vi "play_auto_id.vi"(3 "output-file":path=path "C:/Users/arnold/Documents/afm-cs/labview/first_res_fit_current.json", 4 "time-series-in":refnum<vi>, 6 "Bode amplitude_in":refnum<vi>, 8 "error in":errorcluster, 10 "Amplitude":dbl=0.1 format="%#_13g", 11 "Swept-Sines-Control-Settings":cluster{"u-max":sgl, "offset":sgl, "Ki":sgl}={"u-max"=1.0, "offset"=0.1, "Ki"=0.0}) -> (0 "error out":errorcluster, 1 "Is-Totally-Stable":bool, 2 "auto_id_result":T1)   [LabVIEW 2017]
uses:
  controls/SS_SweptSines.ctl
  controls/SS_sin_params.ctl
  controls/SS_input_data_json.ctl
  controls/fit_sos_results.ctl
  controls/auto_id_result.ctl
  controls/SOS_frf_data.ctl
  controls/logging_selection.ctl
  controls/SS_figures_withtime.ctl
  controls/bode_figure.ctl
  labview/sysID/controls/time_series_figures.ctl
  <vilib>/Utility/error.llb/DialogType.ctl
  <vilib>/FPGAPlugInAG/cRIO-9082/niLvFpga_Open_cRIO-9082.vi
  <vilib>/rvi/interface/common/dynamic/niFpgaDynamicAddResources.vi
  <vilib>/FPGAPlugInAG/Dynamic/niLvFpga_Reset_Dynamic.vi
  <vilib>/rvi/interface/common/niFpgaWaitOnOcc.vi
  <vilib>/Utility/error.llb/Error Cluster From Error Code.vi
  <vilib>/rvi/errors/niLvFpgaAdjustHostInterfaceError.vi
  <vilib>/FPGAPlugInAG/Dynamic/niLvFpga_Run_Dynamic.vi
  <vilib>/FPGAPlugInAG/Dynamic/niLvFpga_Close_Dynamic.vi
  <vilib>/rvi/interface/nirviOpenFPGA/nirviOpenFPGA.xnode
  FPGA Bitfiles/afmimagingcontro_FPGATargetSPARTA_SSfpgasweptsines_lpZqvyn1KNg.lvbitx
  <vilib>/rvi/interface/nirviMethod/nirviMethod.xnode
  <vilib>/rvi/interface/nirviReadWriteControl/nirviReadWriteControl.xnode
  <vilib>/rvi/interface/nirviCloseFPGA/nirviCloseFPGA.xnode
  labview/utils_lib/utils.lvlib
  NiFpgaLv.dll
  <vilib>/rvi/interface/Simulation/niFpgaSimulationCallBeginRW.vi
  <vilib>/addons/_JKI.lib/Serialization/JSON/JKI JSON Serialization.lvlib
  <vilib>/FPGAPlugInAG/Dynamic/niLvFpga_ConfigureFifo_Dynamic.vi
  <vilib>/rvi/errors/niLvFpgaMergeErrorWithErrorCode.vi
panel:
  in  "Tab Control":enum32{"Page 1", "debug", "hide"}(tab)
  in  "control-xy-to-zero":bool=TRUE
  in  "ABORT":bool
  out "fit_sos_result":T3
  in  "theta0":dbl[](array[numeric])=[0.6786, -1.9959, 0.99891, -1.996142, 0.9989]
  out "theta-fit":dbl[](array[numeric])
  out "Bode amplitude":cluster{"W":dbl[], "Magnitude":dbl[]}[](graph) caption="Magnitude Graph"
  in  "Input File (json)":path=path "Z:/afm-cs/sysID/z-axis_sines_info_quick_firstRes.json"
  in  "Figures":enum32{"all-channels", "channel-1", "channel2"}(tab)
  out "Channel 1":cluster{"W":dbl[], "Magnitude":dbl[]}[](graph) caption="Magnitude Graph"
  in  "subtract-mean":bool=TRUE
  out "Channel1 2":cluster{"W":dbl[], "Phase":dbl[]}[](graph) caption="Phase Graph"
  out "Channel 3":cluster{"W":dbl[], "Magnitude":dbl[]}[](graph) caption="Magnitude Graph"
  out "boolean  indicators":T4
  out "Freqs Done":i32(slide) scale=0.0..50.0
  out "number_of_freqs":i32
  out "freq_adjusted":dbl
  out "NaN/Path/Refnum?":bool
  in  "SweptSines (in)":T5={"Log-Channel_select"=[FALSE, FALSE, FALSE, FALSE, FALSE, FALSE], "JSON Header"="", "SS-Params-Array"=[], "input_frequency_definitions"={"Amp"=0.0, "Ts"=0.0, "num_periodsMT"=[], "freqs_Hz"=[], "numAve_s"=[], "Nsamp_total"=[], "Nsettle_s"=[], "Ncollect_s"=[]}, "DAC-ADC primary 2"=0, "Channel-Names"=[], "num_chan"=0, "num-freqs"=0, "Input File (json)"=path "Z:/afm-cs/sysID/x-axis_sines_info_intsamps_quick.json"} {"DAC-ADC primary 2" items=["DAC0/ADC0", "DAC1/ADC1", "DAC2/ADC2", "DAC3/ADC3", ""]}
  out "TsTicks":u32
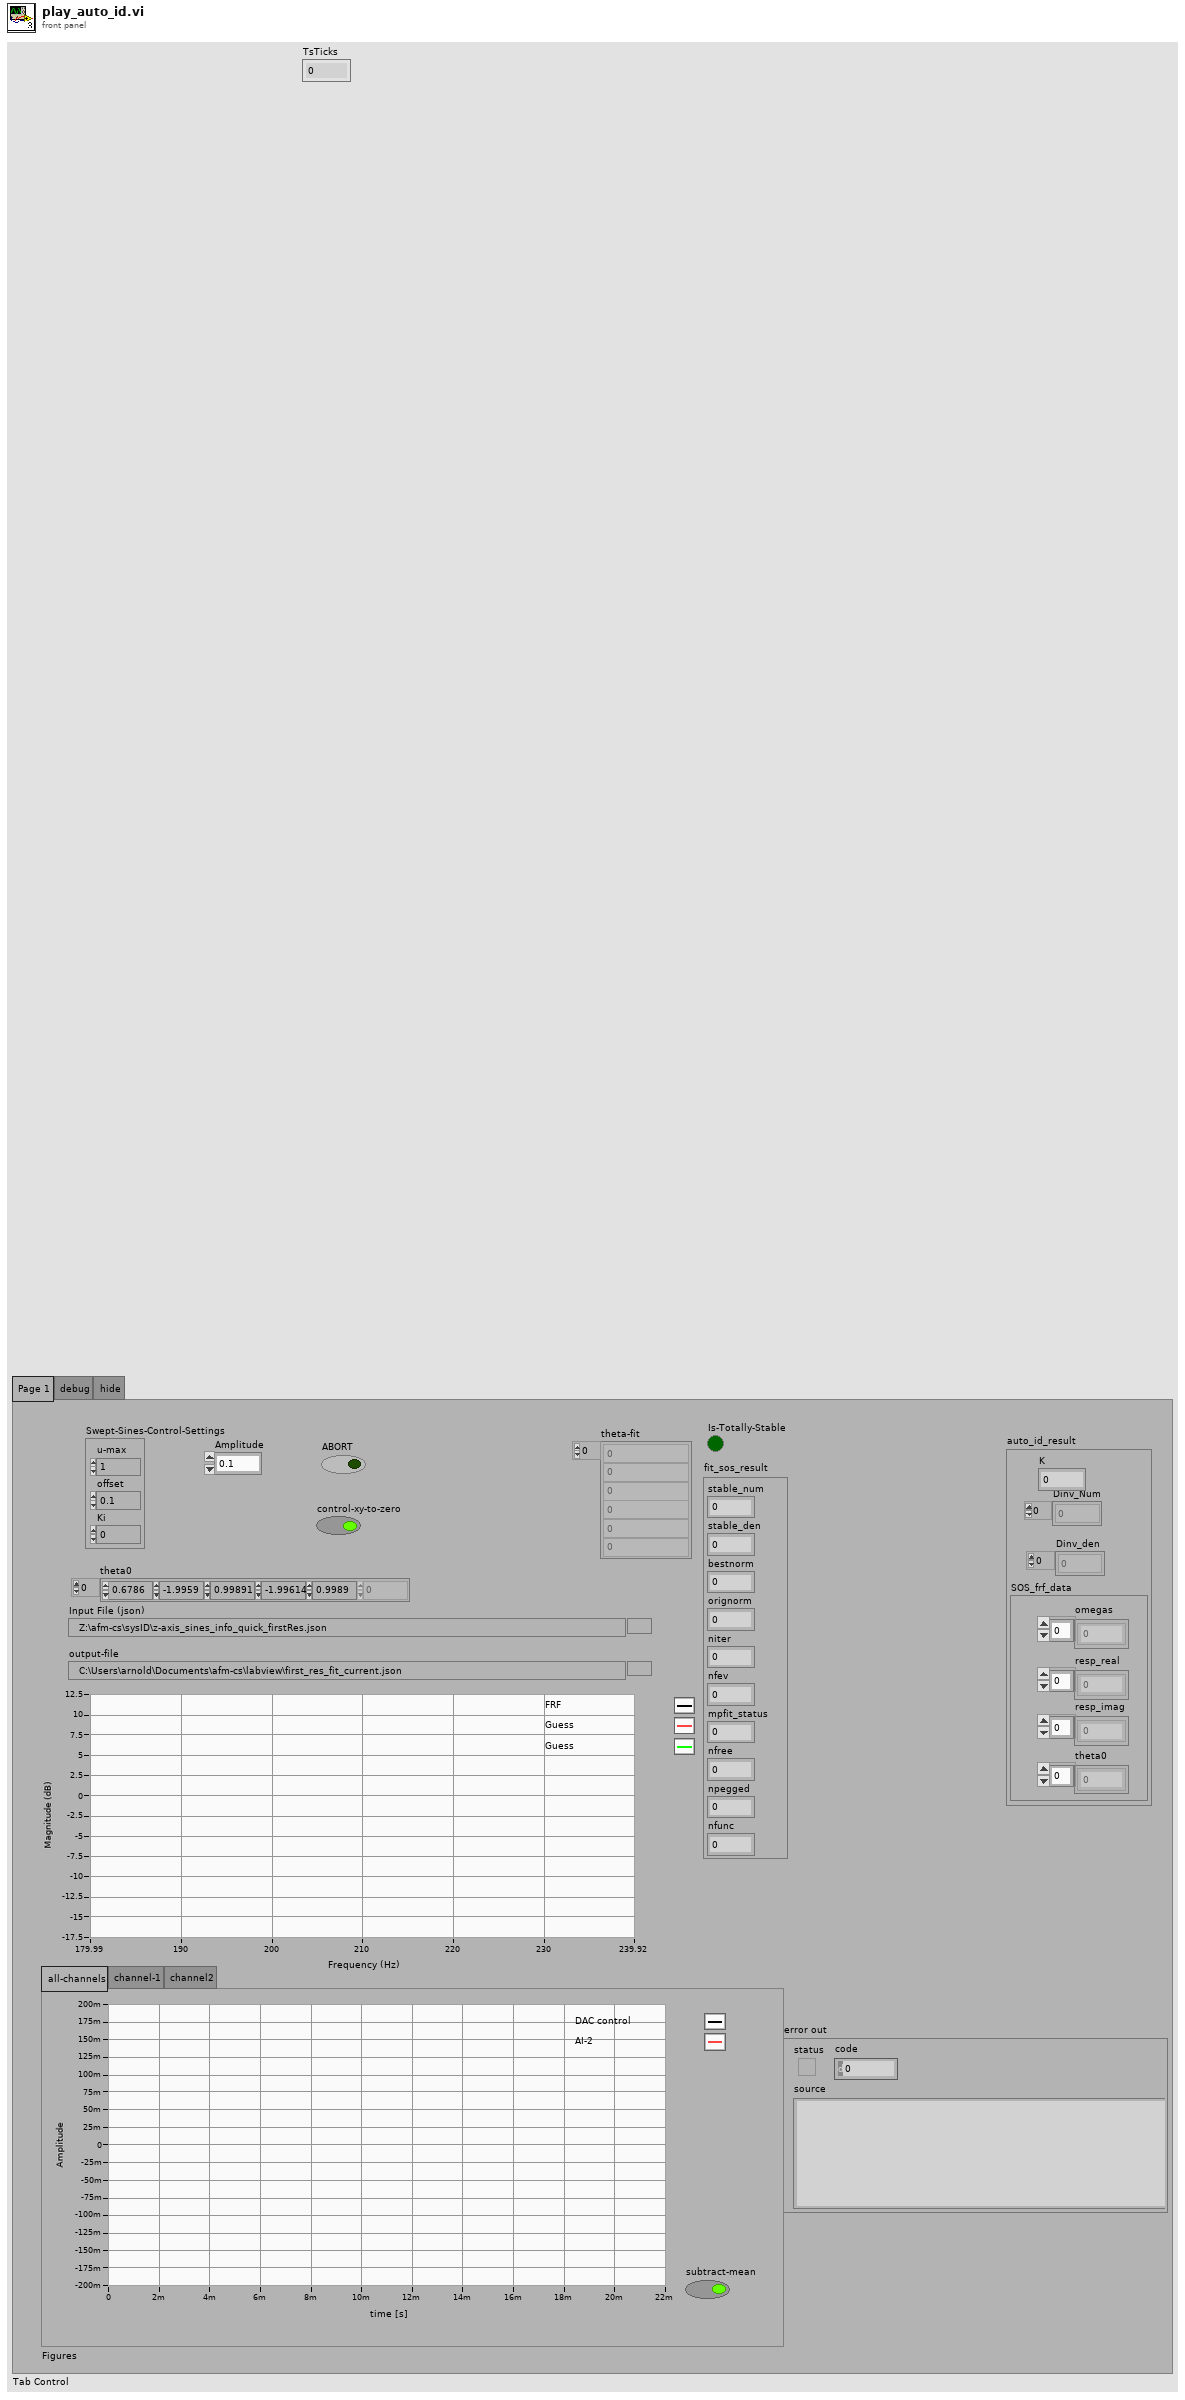
[diagram p1: front panel]
types:
  T1 = typedef "auto_id_result.ctl" = cluster{"Dinv_Num":dbl[], "SOS_frf_data":T2, "Dinv_den":dbl[], "K":dbl}
  T2 = typedef "SOS_frf_data.ctl" = cluster{"omegas":dbl[], "resp_real":dbl[], "resp_imag":dbl[], "theta0":dbl[]}
  T3 = typedef "fit_sos_results.ctl" = cluster{"stable_num":i32, "stable_den":i32, "bestnorm":dbl, "orignorm":dbl, "niter":i32, "nfev":i32, "mpfit_status":i32, "nfree":i32, "npegged":i32, "nfunc":i32}
  T4 = cluster{"unstable-z-traj":bool, "input fifo time-out":bool, "logging fifo timeout":bool, "scanning finished":bool, "unstable-x-traj":bool, "unstable-y-traj":bool, "ABORT":bool, "All Measurements Done":bool, "fpga_finished":bool, "current_scan_finished":bool}
  T5 = typedef "SS_SweptSines.ctl" = cluster{"Log-Channel_select":bool[], "JSON Header":string, "SS-Params-Array":T6[], "input_frequency_definitions":T7, "DAC-ADC primary 2":i16, "Channel-Names":string[], "num_chan":i32, "num-freqs":i32, "Input File (json)":path}
  T6 = typedef "SS_sin_params.ctl" = cluster{"freq":dbl, "num_samples":i32, "Amp":dbl, "Ts":dbl, "N_settle":u32, "Ncollect":i32, "num_periodsMT":i32, "num_averages":i32}
  T7 = typedef "SS_input_data_json.ctl" = cluster{"Amp":dbl, "Ts":dbl, "num_periodsMT":u32[], "freqs_Hz":dbl[], "numAve_s":i32[], "Nsamp_total":u32[], "Nsettle_s":u32[], "Ncollect_s":u32[]}
  T8 = typedef "SS_figures_withtime.ctl" = cluster{"bode figures":T9, "time-series figures":T10, "Freqs Done":refnum<vi>}
  T9 = typedef "bode_figure.ctl" = cluster{"Bode phase":refnum<vi>, "Bode amplitude":refnum<vi>}
  T10 = typedef "time_series_figures.ctl" = refnum<vi>[]
  T11 = typedef "logging_selection.ctl" = cluster{"Collect reference":bool, "Collect DAC control":bool, "Collect AI-0":bool, "Collect AI-1":bool, "Collect AI-2":bool, "Collect AI-3":bool}
  T12 = typedef "FrdData.ctl" = cluster{"Frequency Unit":enum16{"Hz", "rad/s"}, "W":dbl[], "MagDB":dbl[], "PhaseDeg":dbl[], "Resp":cdb[], "Data-name":string}
  T13 = typedef "DialogType.ctl" = u16
  T14 = typedef "SS_experimental-data.ctl" = cluster{"sin-data-out":dbl[][], "Fourier Data":T15, "freq_adjusted?":dbl, "below-nyquist":bool}
  T15 = typedef "SS_FourierData.ctl" = cluster{"E_s":dbl[], "Fourier Coefs":cdb[], "freq-adjusted":dbl}
  T16 = enum16{"open", "replace", "create", "open or create", "replace or create", "replace or create with confirmation"}
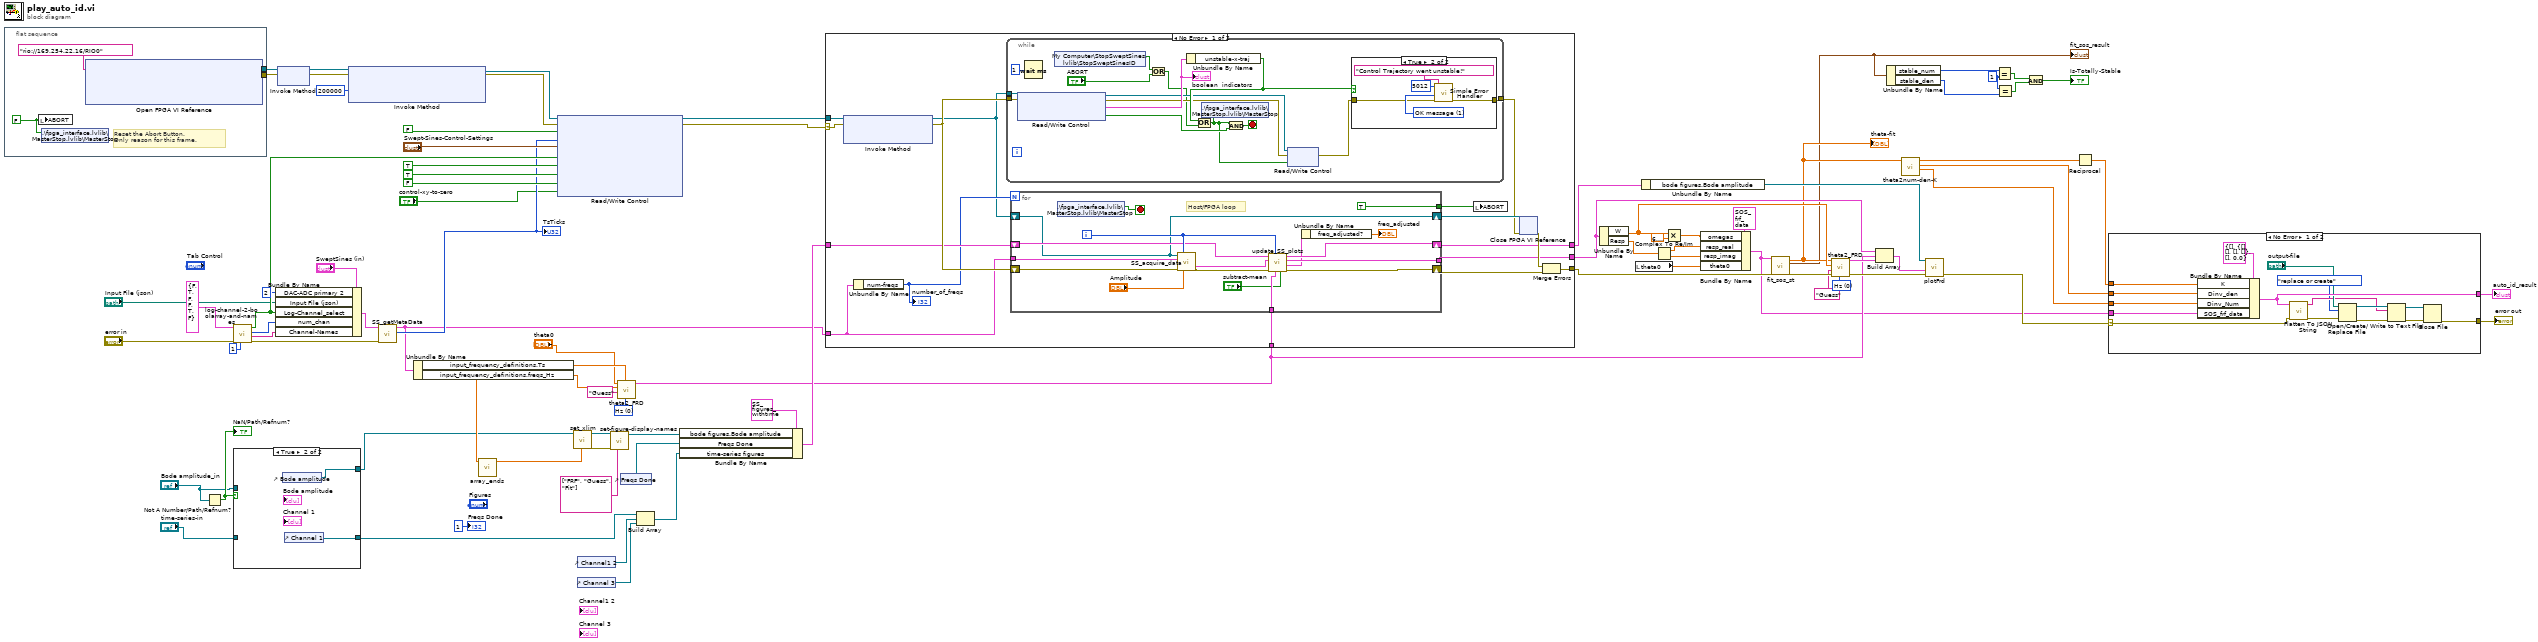
[diagram p0: block diagram]
diagram:
  w23 = 1
  w48 = u16 0 items=["Hz", "rad/s"] ("freq unit")
  w56 = u16 0 items=["Hz", "rad/s"] ("freq unit")
  n1 = flat-sequence {
    tunnel: [w88] -> w84
    tunnel: [w87] -> w83
    frame #0 {
      w86 = FALSE
      # "Reset the Abort Button.\nOnly reason for this frame."
      n2 = local write "ABORT"(w86) -> ()
      n3 = shared-variable ".\\fpga_interface.lvlib\\MasterStop.lvlib\\MasterStop"(w86) -> ()  [unwired: 1 in, 1 out]
      n4 = xnode "Open FPGA VI Reference"("resource name"=tag "rio://169.254.22.16/RIO0") -> ("FPGA VI Reference Out"=w88:refnum<k20>, "error out"=w87:errorcluster)  [unwired: 1 in]
    }
  }
  n5 = Not A Number/Path/Refnum?(number/path/refnum="Bode amplitude_in") -> (NaN/Path/Refnum?=w5:bool)
  "NaN/Path/Refnum?" <- w5
  n6 = call "log-channel-2-boolarray-and-names.vi"("min_number_chan"=i16 1, "error in"="error in", "Logging selection"=T11 {"Collect reference"=FALSE, "Collect DAC control"=TRUE, "Collect AI-0"=FALSE, "Collect AI-1"=FALSE, "Collect AI-2"=TRUE, "Collect AI-3"=FALSE}) -> ("error out"=w72:errorcluster, "Channel-Names"=w70:string[], "num_chan"=w67:i32, "Log-Channel_select"=w65:bool[])  [unwired: 5 in]
  n7 = case shown="True" w5 {
    tunnel: [w91 w93] -> w3
    tunnel: "Bode amplitude_in" -> [w91 _]
    tunnel: [w90 w92] -> w2
    tunnel: "time-series-in" -> [w90 _]
    frame False {
    }
    frame True {
      n8 = control-ref of="Bode amplitude"() -> (w93:refnum<vi>)
      n9 = control-ref of="Channel 1"() -> (w92:refnum<vi>)
    }
  }
  n10 = Bundle By Name(cluster="SweptSines (in)", "DAC-ADC primary 2"=i16 2, "Input File (json)"="Input File (json)", "Log-Channel_select"=w65, "num_chan"=w67, "Channel-Names"=w70) -> (w69:T5)
  n11 = xnode "Invoke Method"("FPGA VI Reference In"=w84, "error in"=w83) -> ("FPGA VI Reference Out"=w77:refnum<k20>, "error out"=w76:errorcluster)
  n12 = xnode "Invoke Method"("FPGA VI Reference In"=w77, "error in"=w76, "Requested Depth"=200000 ("requested depth")) -> ("FPGA VI Reference Out"=w82:refnum<k20>, "error out"=w78:errorcluster)  [unwired: 1 out]
  n13 = call "SS_getMetaData.vi"("error in"=w72, "SweptSines"=w69) -> ("TsTicks"=w62:u32, "SweptSines (out)"=w33:T5)  [unwired: 6 in, 1 out]
  "TsTicks" <- w62
  n14 = Unbundle By Name(w33) -> ("input_frequency_definitions.Ts"=w55:dbl, "input_frequency_definitions.freqs_Hz"=w54:dbl[])
  n15 = call "array_ends.vi"("freqs_Hz"=w54) -> ("Array"=w58:dbl[])  [unwired: 10 in]
  n16 = xnode "Read/Write Control"("FPGA VI Reference In"=w82, "error in"=w78, "ABORT"=FALSE, "TsTicks"=w62, "Swept-Sines-Control-Settings"="Swept-Sines-Control-Settings", "Log-Channel_select"=w65, "Subtract y0?"=TRUE ("Subtract-origin"), "reset"=TRUE, "Close Loop?"=FALSE, "control-xy-zero"="control-xy-to-zero") -> ("FPGA VI Reference Out"=w74:refnum<k20>, "error out"=w73:errorcluster)
  n17 = call "set_xlim.vi"("xlim"=w58, "figure (in)"=w3) -> ("error out"=w59:errorcluster, "figure (out)"=w60:refnum<vi>)  [unwired: 8 in]
  n18 = control-ref of="Channel1 2"() -> (w8:refnum<vi>)
  n19 = control-ref of="Channel 3"() -> (w7:refnum<vi>)
  n20 = call "set-figure-display-names.vi"("DisplayNames"=string[] ["FRF", "Guess", "Fit"] ("Data_names"), "error in"=w59, "figure (in)"=w60) -> ("figure (out)"=w53:refnum<vi>)  [unwired: 7 in, 1 out]
  n21 = call "theta2_FRD.vi"("freq unit"=w56, "Sampling Time (s)"=w55, "Data-name"="Guess", "freqs/omega"=w54, "theta"="theta0") -> ("FRD-model"=w34:T12)  [unwired: 5 in, 1 out]
  n22 = control-ref of="Freqs Done"() -> (w29:refnum<vi>)
  n23 = Build Array(w2, w8, w7) -> (w6:refnum<vi>[])
  n24 = Bundle By Name(cluster=T8 {"bode figures"={"Bode phase"=refnum, "Bode amplitude"=refnum}, "time-series figures"=[], "Freqs Done"=refnum} ("figures"), "bode figures.Bode amplitude"=w53, "Freqs Done"=w29, "time-series figures"=w6) -> (w52:T8)
  n25 = case shown="No Error" w73 {
    selector: w73 -> [w99 w149]
    tunnel: w74 -> [w109 _]
    tunnel: [w104 w149] -> w61
    tunnel: w33 -> [w101 _]
    tunnel: w52 -> [w102 w148]
    tunnel: [w97 w148] -> w40
    tunnel: w34 -> [w96 _]
    tunnel: [w95 _] -> w35
    frame No Error {
      n26 = xnode "Invoke Method"("FPGA VI Reference In"=w109, "error in"=w99) -> ("FPGA VI Reference Out"=w94:refnum<k20>, "error out"=w107:errorcluster)  [unwired: 1 in]
      n27 = Unbundle By Name(w101) -> ("num-freqs"=w100:i32)
      "number_of_freqs" <- w100
      n28 = while {
        tunnel: w94 -> [w123]
        tunnel: w107 -> [w122]
        tunnel: [w119] -> w103
        stop <- w115 stop-if-true
        n29 = xnode "Read/Write Control"("FPGA VI Reference In"=w123, "error in"=w122) -> ("FPGA VI Reference Out"=w118:refnum<k20>, "error out"=w117:errorcluster, "boolean  indicators"=w121:T4, "All Done"=w114:bool)
        "boolean  indicators" <- w121
        n30 = Wait (ms)(milliseconds to wait=u32 1) -> ()  [unwired: 1 out]
        n31 = shared-variable "My Computer\\StopSweptSines.lvlib\\StopSweptSinesID"() -> (w110:bool)  [unwired: 1 in, 1 out]
        n32 = Or(x=w110, y="ABORT") -> (x .or. y?=w111:bool)
        n33 = Unbundle By Name(w121) -> ("unstable-x-traj"=w120:bool)
        n34 = Or(x=w120, y=w111) -> (x .or. y?=w113:bool)
        n35 = shared-variable ".\\fpga_interface.lvlib\\MasterStop.lvlib\\MasterStop"(w113) -> ()  [unwired: 1 in, 1 out]
        n36 = And(x=w113, y=w114) -> (x .and. y?=w115:bool)
        n37 = xnode "Read/Write Control"("FPGA VI Reference In"=w118, "error in"=w117, "ABORT"=w113) -> ("error out"=w116:errorcluster)  [unwired: 1 out]
        n38 = case shown="True" w120 {
          tunnel: w116 -> [w125 w127]
          tunnel: [w125 w126] -> w119
          frame False {
          }
          frame True {
            w130 = T13 1 items=["no dialog", "OK message", "continue or stop message", "OK message + warnings", "continue/stop + warnings"] ("type of dialog (OK msg:1)")
            n39 = call <vilib>:"Simple Error Handler.vi"("error code (no error:0)"=5012, "error source (\" \")"="Control Trajectory went unstable!" ("error source (\" \")"), "type of dialog (OK msg:1)"=w130, "error in (no error)"=w127) -> ("error out"=w126:errorcluster)  [unwired: 1 in, 4 out]
          }
        }
      }
      n40 = for {
        N: w100 -> [_]
        shift-right: [w137] -> w97
        shift-left: w102 -> [w136]
        tunnel: [TRUE] -> w106
        shift-right: [w143] -> w98
        shift-left: w107 -> [w145]
        tunnel: w101 -> [w144]
        tunnel: [w138] -> w95
        tunnel: w96 -> [w134]
        shift-right: [w132] -> w108
        shift-left: w94 -> [w132]
        i -> [w141]
        stop <- w133 stop-if-true
        # "Host/FPGA loop"
        n41 = shared-variable ".\\fpga_interface.lvlib\\MasterStop.lvlib\\MasterStop"() -> (w133:bool)  [unwired: 1 in, 1 out]
        n42 = call "SS_acquire_data.vi"("Type"=w132, "idx"=w141, "SweptSines (in)"=w144, "error in"=w145, "Signal Amplitude (V)"="Amplitude") -> ("experiment-data"=w140:T14, "error IO"=w139:errorcluster)  [unwired: 7 in, 2 out]
        n43 = call "update_SS_plots.vi"("subtract-mean"="subtract-mean", "other-frd"=w134, "freqs-iter"=w141, "error in (no error)"=w139, "experiment-data"=w140, "figures-in"=w136) -> ("error out"=w143:errorcluster, "experiment-data (out)"=w135:T14, "FRD-out"=w138:T12, "figures-out"=w137:T8)  [unwired: 2 in]
        n44 = Unbundle By Name(w135) -> ("freq_adjusted?"=→"freq_adjusted":dbl)
      }
      n45 = local write "ABORT"(w106) -> ()
      n46 = xnode "Close FPGA VI Reference"("FPGA VI Reference In"=w108, "error in"=w103) -> ("error out"=w105:errorcluster)
      n47 = Merge Errors(w105, w98) -> (w104:errorcluster)
    }
    frame Error {
    }
  }
  n48 = Unbundle By Name(w35) -> ("W"=w28:dbl[], "Resp"=w42:cdb[])
  n49 = local read "theta0"() -> (w41:dbl[])
  n50 = Unbundle By Name(w40) -> ("bode figures.Bode amplitude"=w36:refnum<vi>)
  n51 = Complex To Re/Im(x + iy=w42) -> (x=w44:dbl[], y=w43:dbl[])
  n52 = Multiply(x=w28, y=6.283185307179586) -> (x*y=w46:dbl[])
  n53 = Bundle By Name(cluster=T2 {"omegas"=[1006.674891, 1016.262272, 1025.849652, 1035.437033, 1045.024413, 1054.611794, 1064.199174, 1073.786548, 1083.373929, 1092.961309, 1102.54869, 1112.13607, 1121.723451, 1131.310831, 1140.898212, 1150.485592, 1160.072973, 1169.660354, 1179.247728, 1188.835108, 1198.422489, 1208.009869, 1217.59725, 1227.18463, 1236.772011, 1246.359391, 1255.946772, 1265.534152, 1275.121533, 1284.708907, 1294.296288, 1303.883668, 1313.471049, 1323.058429, 1332.64581, 1342.23319, 1351.820571, 1361.407951, 1370.995332, 1380.582706, 1390.170086, 1399.757467, 1409.344847, 1418.932228, 1428.519609, 1438.106989, 1447.69437, 1457.28175, 1466.869131, 1476.456511, 1486.043885, 1495.631266, 1505.218646, 1514.806027, 1524.393407, 1533.980788, 1543.568168, 1553.155549, 1562.742929, 1572.33031, 1581.91769, 1591.505065, 1601.092445, 1610.679826, 1620.267206, 1629.854587, 1639.441967, 1649.029348, 1658.616728], "resp_real"=[0.6710936201, 0.6732167298, 0.6736550301, 0.6739624194, 0.6764113406, 0.6760996891, 0.6752809587, 0.67695858, 0.6764911126, 0.6818501379, 0.6804259731, 0.6777421689, 0.683602427, 0.6839502494, 0.6873055899, 0.6871681129, 0.6836241729, 0.6933718335, 0.6965190689, 0.7011525702, 0.7041006273, 0.7087951209, 0.7138881005, 0.7230810664, 0.7347158563, 0.743593779, 0.7581554602, 0.7740064901, 0.7983882262, 0.8168799192, 0.8500537495, 0.885993569, 0.8534751304, 0.6135298299, 0.1963078728, 0.06997493602, 0.2143720387, 0.3262401307, 0.3874363268, 0.4244315327, 0.4518076771, 0.4783094111, 0.4942330365, 0.5078067569, 0.5183774173, 0.5254372068, 0.5346584888, 0.5422376, 0.5476692529, 0.546204086, 0.5501300272, 0.5526801006, 0.557631838, 0.5639162136, 0.5601299408, 0.5627301292, 0.5646599194, 0.5678509651, 0.5674161925, 0.5676099823, 0.5703128211, 0.5717199117, 0.5717616028, 0.5714305364, 0.5706488864, 0.574491682, 0.5720673373, 0.5722619255, 0.5727540208], "resp_imag"=[0.1828230252, 0.185702312, 0.1893108783, 0.1927179342, 0.1939516982, 0.1991804891, 0.1996588255, 0.1997489381, 0.2009184192, 0.2058333084, 0.205968755, 0.2071290225, 0.2120033665, 0.2140896781, 0.2197333799, 0.2218060221, 0.2270970718, 0.2243543787, 0.2282290931, 0.2349554807, 0.2362899955, 0.2386023634, 0.2479762836, 0.2514213949, 0.2589829258, 0.2690734156, 0.2817668466, 0.3075000844, 0.3292949756, 0.3581777586, 0.418098085, 0.518537997, 0.7274335428, 0.9954410219, 0.8283414758, 0.4651799029, 0.2632646215, 0.2204933474, 0.2100370796, 0.215817828, 0.2094899805, 0.2041701149, 0.2090161752, 0.2122336611, 0.2144513636, 0.2154505064, 0.2184072105, 0.2207006189, 0.2264320741, 0.2319746485, 0.2352243002, 0.2359211056, 0.2344839067, 0.234200787, 0.2350554818, 0.2419460399, 0.2451480379, 0.2422561944, 0.2450402058, 0.2520603413, 0.2526693987, 0.2530329194, 0.2523935129, 0.2570623818, 0.2576871444, 0.2563998974, 0.259830217, 0.2610581842, 0.2647075477], "theta0"=[0.6786, -1.9959, 0.99891, -1.996142, 0.9989]} ("SOS-frf_data"), "omegas"=w46, "resp_real"=w44, "resp_imag"=w43, "theta0"=w41) -> (w16:T2)
  n54 = call "fit_sos_st.vi"("frf_data"=w16, "error in (no error)"=w61) -> ("theta"=w27:dbl[], "fit_sos_result"=w26:T3, "error out"=w50:errorcluster)  [unwired: 23 in]
  "fit_sos_result" <- w26
  "theta-fit" <- w27
  n55 = call "theta2_FRD.vi"("freq unit"=w48, "error in (no error)"=w50, "Data-name"="Guess", "freqs/omega"=w28, "theta"=w27) -> ("error out"=w37:errorcluster, "FRD-model"=w39:T12)  [unwired: 5 in]
  n56 = Build Array(w35, w34, w39) -> (w38:T12[])
  n57 = Unbundle By Name(w26) -> ("stable_num"=w25:i32, "stable_den"=w24:i32)
  n58 = call "theta2num-den-K.vi"("theta"=w27) -> ("Den"=w12:dbl[], "Num"=w17:dbl[], "K"=w11:dbl)  [unwired: 8 in]
  n59 = call "plotFrd.vi"("error in (no error)"=w37, "FRD-array"=w38, "Magnitude Graph Reference in"=w36) -> ("error out"=w18:errorcluster)  [unwired: 6 in, 2 out]
  n60 = Equal?(x=w25, y=w23) -> (x = y?=w21:bool)
  n61 = Equal?(x=w23, y=w24) -> (x = y?=w22:bool)
  n62 = And(x=w21, y=w22) -> (x .and. y?=→"Is-Totally-Stable":bool)
  n63 = Reciprocal(x=w11) -> (1/x=w10:dbl)
  n64 = case shown="No Error" w18 {
    selector: w18 -> [w161 w166]
    tunnel: w12 -> [w164 _]
    tunnel: w17 -> [w163 _]
    tunnel: w16 -> [w162 _]
    tunnel: [w153 w166] -> w14
    tunnel: [w160 _] -> w15
    tunnel: w10 -> [w150 _]
    frame No Error {
      n65 = Bundle By Name(cluster=T1 {"Dinv_Num"=[], "SOS_frf_data"={"omegas"=[], "resp_real"=[], "resp_imag"=[], "theta0"=[]}, "Dinv_den"=[], "K"=0.0} ("auto_id_result 2"), "K"=w150, "Dinv_den"=w163, "Dinv_Num"=w164, "SOS_frf_data"=w162) -> (w160:T1)
      n66 = call <vilib>:"Flatten To JSON String.vi"("error in (no error)"=w161, "Variant"=w160) -> ("error out"=w158:errorcluster, "JSON String"=w155:string)  [unwired: 8 in]
      n67 = Open/Create/Replace File(file path (use dialog)="output-file", error in=w158, operation (0:open)=T16."replace or create") -> (refnum out=w159:refnum<file>, error out=w157:errorcluster)  [unwired: 3 in, 1 out]
      n68 = Write to Text File(file (use dialog)=w159, text=w155, error in=w157) -> (refnum out=w152:refnum<file>, error out=w154:errorcluster)  [unwired: 1 in, 1 out]
      n69 = Close File(refnum=w152, error in=w154) -> (error out=w153:errorcluster)  [unwired: 1 out]
    }
    frame Error {
    }
  }
  "error out" <- w14
  "auto_id_result" <- w15
  "Freqs Done" <- 1 ("Freqs Done")
